vi "traffic signal.vi"() -> ()   [LabVIEW 2018]
panel:
  out "Boolean 3":bool
  out "Boolean 2":bool
  out "Boolean":bool
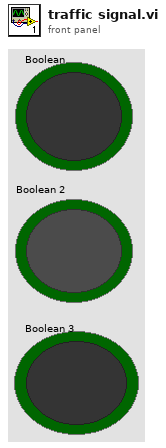
[diagram p1: front panel]
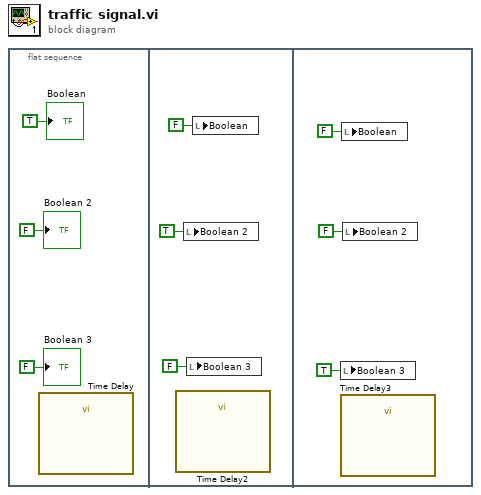
[diagram p0: block diagram]
diagram:
  n1 = flat-sequence {
    frame #0 {
      n2 = call "Time Delay"() -> ()  [unwired: 11 in, 1 out]
      "Boolean" <- TRUE ("Boolean")
      "Boolean 2" <- FALSE ("Boolean 2")
      "Boolean 3" <- FALSE ("Boolean 3")
    }
    frame #1 {
      n3 = call "Time Delay2"() -> ()  [unwired: 11 in, 1 out]
      n4 = local write "Boolean 2"(TRUE ("Boolean 2")) -> ()
      n5 = local write "Boolean 3"(FALSE ("Boolean 3")) -> ()
      n6 = local write "Boolean"(FALSE ("Boolean")) -> ()
    }
    frame #2 {
      n7 = local write "Boolean 3"(TRUE ("Boolean 3")) -> ()
      n8 = call "Time Delay3"() -> ()  [unwired: 11 in, 1 out]
      n9 = local write "Boolean"(FALSE ("Boolean")) -> ()
      n10 = local write "Boolean 2"(FALSE ("Boolean 2")) -> ()
    }
  }
